vi "target.vi"() -> ()   [LabVIEW 2020]
uses:
  <vilib>/rvi/interface/RandomDataEmulation/niFpgaRandomDataHandleErrors.vi
  <vilib>/rvi/DataTransferAndStorage/Container/XNode/niFpgaContainer.xnode
  <vilib>/rvi/interface/RandomDataEmulation/nirviRandomDataFpgaReadWriteTemplate.vi
panel:
  out "n":i32
  out "m":i32
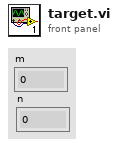
[diagram p1: front panel]
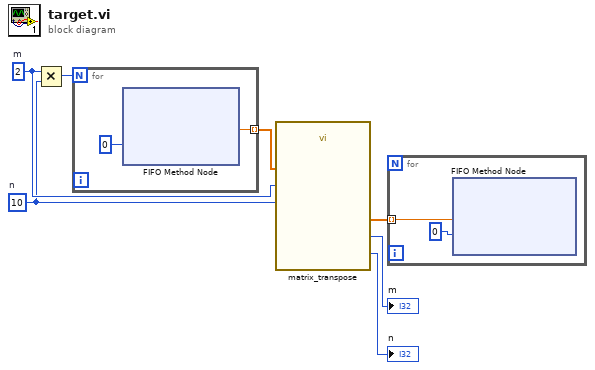
[diagram p0: block diagram]
diagram:
  w5 = 10  # n
  w6 = 2  # m
  n1 = Multiply(x=w6, y=w5) -> (x*y=w3:i32)
  n2 = for {
    N: w3 -> [_]
    tunnel: [w9] -> w7 mode=indexing
    n3 = xnode ("FIFO Method Node")("Timeout"=0) -> ("Element"=w9:sgl)  [unwired: 1 in, 2 out]
  }
  n4 = call "matrix_transpose.vi"("n"=w5, "m"=w6, "A"=w7) -> ("n"=→"n":i32, "m"=→"m":i32, "B"=w4:sgl[])
  n5 = for {
    tunnel: w4 -> [w11] mode=indexing
    n6 = xnode ("FIFO Method Node")("Element"=w11, "Timeout"=0) -> ()  [unwired: 1 in, 2 out]
  }
